vi "ArrayFile.vi"(10 "n":i32, 11 "File Path":string) -> (2 "error out":errorcluster caption="에러 출력", 3 "Array":dbl[](array[numeric]))   [LabVIEW 2014]
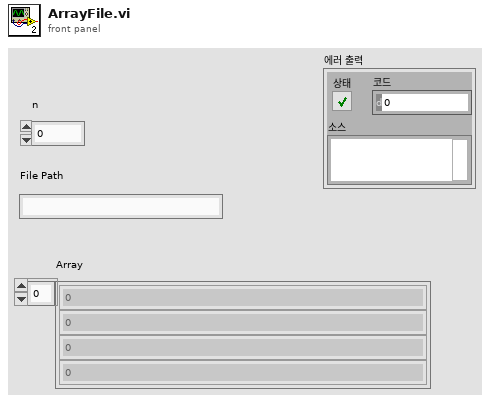
[diagram p1: front panel]
types:
  T1 = enum16{"open", "replace", "create", "open or create", "replace or create", "replace or create with confirmation"}
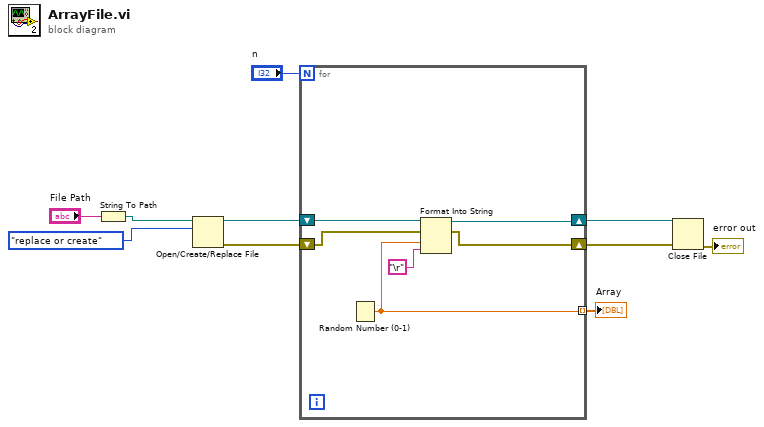
[diagram p0: block diagram]
diagram:
  n1 = String To Path(string="File Path") -> (path=w9:path)
  n2 = Open/Create/Replace File(file path (use dialog)=w9, operation (0:open)=T1."replace or create" ("동작(0:open)")) -> (refnum out=w7:refnum<file>, error out=w4:errorcluster)  [unwired: 4 in, 1 out]
  n3 = for {
    N: "n" -> [_]
    shift-right: [w15] -> w6
    shift-left: w7 -> [w16]
    shift-right: [w13] -> w3
    shift-left: w4 -> [w14]
    tunnel: [w12] -> w2 mode=indexing
    n4 = Random Number (0-1)() -> (number: 0 to 1=w12:dbl)
    n5 = Format Into String(initial string=w16, error in=w14, w12, "\r") -> (resulting string=w15:refnum<file>, error out=w13:errorcluster)  [unwired: 1 in]
  }
  "Array" <- w2
  n6 = Close File(refnum=w6, error in=w3) -> (error out=→"error out":errorcluster)  [unwired: 1 out]
